vi "ConvertSENIndextoSensitivityString.vi"(8 "error in (no error)":errorcluster, 9 "IMODE":string, 10 "SEN":string) -> (0 "error out":errorcluster, 1 "Sensitivity (A or V)":dbl, 2 "Sensitivty":string)   [LabVIEW 2016, in "SR7270 Drivers.lvlib"]
uses:
  SR7270 Drivers.lvlib
  Typedefs/SEN-IMODE1--enum.ctl
  Typedefs/SEN-IMODE2--enum.ctl
  Typedefs/SEN-IMODE0--enum.ctl
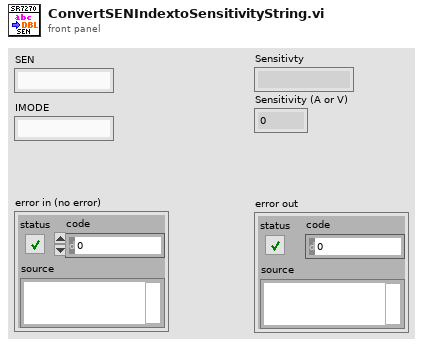
[diagram p1: front panel]
types:
  T1 = typedef "SR7270 Drivers.lvlib/SEN-IMODE0--enum.ctl" = enum16{"2 nV", "5 nV", "10 nV", "20 nV", "50 nV", "100 nV", "200 nV", "500 nV", "1 µV", "2 µV", "5 µV", "10 µV", "20 µV", "50 µV", "100 µV", "200 µV", "500 µV", "1 mV", "2 mV", "5 mV", "10 mV", "20 mV", "50 mV", "100 mV", "200 mV", "500 mV", "1 V"}
  T2 = typedef "SR7270 Drivers.lvlib/SEN-IMODE2--enum.ctl" = enum16{"2 fA", "5 fA", "10 fA", "20 fA", "50 fA", "100 fA", "200 fA", "500 fA", "1 pA", "2 pA", "5 pA", "10 pA", "20 pA", "50 pA", "100 pA", "200 pA", "500 pA", "1 nA", "2 nA", "5 nA", "10 nA"}
  T3 = typedef "SR7270 Drivers.lvlib/SEN-IMODE1--enum.ctl" = enum16{"2 fA", "5 fA", "10 fA", "20 fA", "50 fA", "100 fA", "200 fA", "500 fA", "1 pA", "2 pA", "5 pA", "10 pA", "20 pA", "50 pA", "100 pA", "200 pA", "500 pA", "1 nA", "2 nA", "5 nA", "10 nA", "20 nA", "50 nA", "100 nA", "200 nA", "500 nA", "1 µA"}
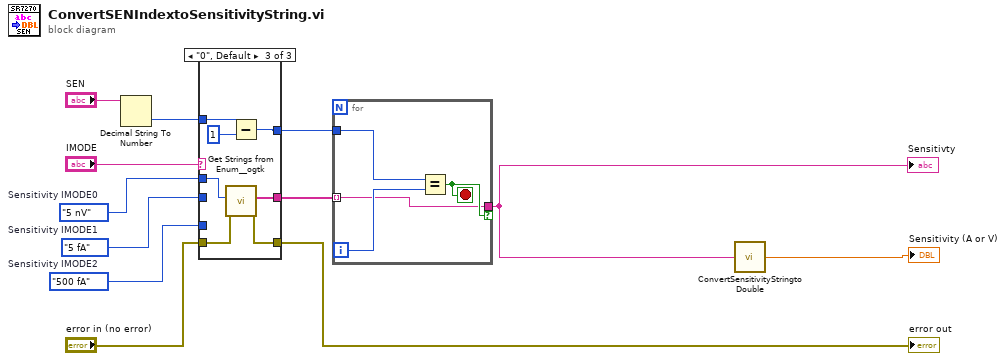
[diagram p0: block diagram]
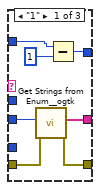
[diagram p2: hidden frame]
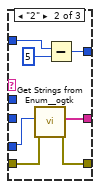
[diagram p3: hidden frame]
diagram:
  w9 = SEN-IMODE0--enum."5 nV"  # Sensitivity IMODE0
  w7 = SEN-IMODE2--enum."500 fA"  # Sensitivity IMODE2
  w8 = SEN-IMODE1--enum."5 fA"  # Sensitivity IMODE1
  n1 = Decimal String To Number(string="SEN") -> (number=w6:i32)  [unwired: 2 in, 1 out]
  n2 = case shown="\"0\", Default" "IMODE" {
    tunnel: w9 -> [_ _ w30]
    tunnel: w8 -> [w16 _ _]
    tunnel: w7 -> [_ w23 _]
    tunnel: w6 -> [w18 w25 w32]
    tunnel: [w17 w24 w31] -> w5
    tunnel: [w15 w22 w29] -> w3
    tunnel: "error in (no error)" -> [w14 w21 w28]
    tunnel: [w13 w20 w27] -> w1
    frame "1" {
      n3 = call <userlib>:"Get Strings from Enum__ogtk.vi"("error in (no error)"=w14, "Enum"=w16) -> ("error out"=w13:errorcluster, "Enum Strings"=w15:string[])  [unwired: 6 in, 2 out]
      n4 = Subtract(x=w18, y=1) -> (x-y=w17:i32)
    }
    frame "2" {
      n5 = call <userlib>:"Get Strings from Enum__ogtk.vi"("error in (no error)"=w21, "Enum"=w23) -> ("error out"=w20:errorcluster, "Enum Strings"=w22:string[])  [unwired: 6 in, 2 out]
      n6 = Subtract(x=w25, y=5) -> (x-y=w24:i32)
    }
    frame "0", Default {
      n7 = call <userlib>:"Get Strings from Enum__ogtk.vi"("error in (no error)"=w28, "Enum"=w30) -> ("error out"=w27:errorcluster, "Enum Strings"=w29:string[])  [unwired: 6 in, 2 out]
      n8 = Subtract(x=w32, y=1) -> (x-y=w31:i32)
    }
  }
  "error out" <- w1
  n9 = for {
    tunnel: [w34] -> w4 if=w37
    tunnel: w3 -> [w34] mode=indexing
    tunnel: w5 -> [w36]
    i -> [w35]
    stop <- w37 stop-if-true
    n10 = Equal?(x=w36, y=w35) -> (x = y?=w37:bool)
  }
  "Sensitivty" <- w4
  n11 = call "ConvertSensitivityStringtoDouble.vi"("Sensitivity"=w4) -> ("Sensitivtiy"=→"Sensitivity (A or V)":dbl)
